vi "分贝计算.vi"(11 "数组":dbl[](array[numeric])) -> (3 "数值":dbl)   [LabVIEW 2011]
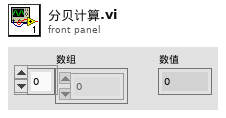
[diagram p1: front panel]
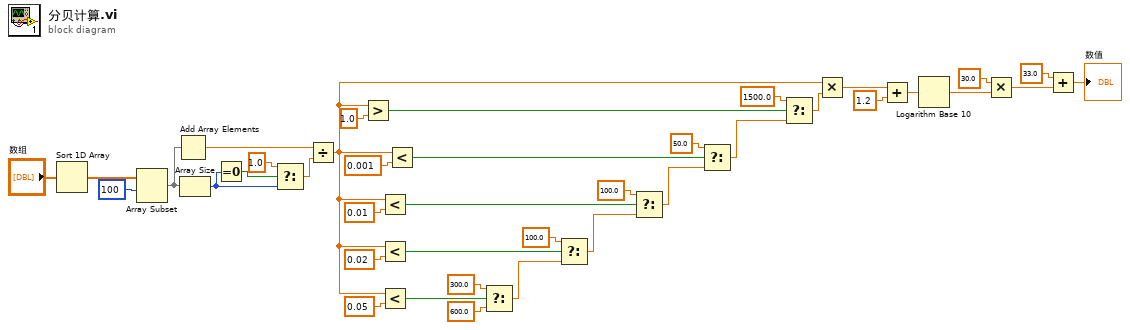
[diagram p0: block diagram]
diagram:
  n1 = Sort 1D Array(array="数组") -> (sorted array=w10:dbl[])
  n2 = Array Subset(array=w10, index=100 ("索引")) -> (w16:dbl[])  [unwired: 1 in]
  n3 = Add Array Elements(numeric array=w16) -> (sum=w15:dbl)
  n4 = Array Size(array=w16) -> (size(s)=w1:i32)
  n5 = Equal To 0?(x=w1) -> (x = 0?=w4:bool)
  n6 = Select(t=1.0, s=w4, f=w1) -> (s? t:f=w2:dbl)
  n7 = Divide(x=w15, y=w2) -> (x/y=w36:dbl)
  n8 = Greater?(x=w36, y=1.0) -> (0:w29:bool)
  n9 = Less?(x=w36, y=0.01) -> (x < y?=w21:bool)
  n10 = Less?(x=w36, y=0.02) -> (x < y?=w18:bool)
  n11 = Less?(x=w36, y=0.05) -> (x < y?=w34:bool)
  n12 = Less?(x=w36, y=0.001) -> (x < y?=w25:bool)
  n13 = Select(t=300.0, s=w34, f=600.0) -> (s? t:f=w37:dbl)
  n14 = Select(t=100.0, s=w18, f=w37) -> (s? t:f=w23:dbl)
  n15 = Select(t=100.0, s=w21, f=w23) -> (s? t:f=w27:dbl)
  n16 = Select(t=50.0, s=w25, f=w27) -> (s? t:f=w31:dbl)
  n17 = Select(t=1500.0, s=w29, f=w31) -> (s? t:f=w32:dbl)
  n18 = Multiply(x=w36, y=w32) -> (x*y=w8:dbl)
  n19 = Add(x=w8, y=1.2) -> (x+y=w6:dbl)
  n20 = Logarithm Base 10(1:w6) -> (0:w7:dbl)
  n21 = Multiply(x=30.0, y=w7) -> (x*y=w13:dbl)
  n22 = Add(x=33.0, y=w13) -> (x+y=→"数值":dbl)
